vi "JESD Sync TX.vi"(0 "fpga ref in":T7, 2 "txjesd.LmfcDly":fxp<+,5,5>=2.0, 5 "Board Settings in":T1={"VISA resource name"="", "Address Space"=1, "window_offset"=0, "register_addresses"={"MM based Registers"={"Revision"=0, "OldestCompatRev"=0, "signature"=0, "scratch"=0, "LedControl"=0, "BoardHwRev"=0, "BoardControl"=0, "ThermalStatus"=0, "BasebandStatus"=0, "BasebandControl"=0, "BasebandAuxSetup"=0, "BasebandAuxStatus"=0, "LmkSyncOutSetup"=0, " AdcSyncOutSetup"=0, " InjSyncOutSetup"=0, " PxiTrig0OutSetup"=0, " PxiTrig1OutSetup"=0, " PxiTrig2OutSetup"=0, " PxiTrig3OutSetup"=0, " PxiTrig4OutSetup"=0, " PxiTrig5OutSetup"=0, " PxiTrig6OutSetup"=0, " PxiTrig7OutSetup"=0}, "CPLD based Registers"={"SlaveSignature"=0, "SlaveRevision"=0, "SlaveOldestCompatRev"=0, "SlaveScratch"=0, "SlaveSetup"=0, "SlaveStatus"=0, "IDacReg_offset"=0, "LMKRegGrp0_offset"=0, "QDacReg_offset"=0, "BrdTempSensorVal"=0, "TempSensorPowerDown"=0, "GPIOReg_offset"=0, "IAdcReg_offset"=0, "QAdcReg_offset"=0, "LMKRegGrp1_offset"=0, "QadcTempSensorVal"=0, "IadcTempSensorVal"=0, "RevisionReg"=0, "VcxoReg"=0, "CpldStatusReg"=0, "PowerReg"=0, "VBiasEnReg"=0, "ExtRefOeReg"=0, "QdacCtrlReg"=0, "QdacStatusReg"=0, "IdacCtrlReg"=0, "IdacStatusReg"=0, "QdacJtagIn"=0, "QdacJtagOut"=0, "IdacJtagIn"=0, "IdacJtagOut"=0, "IqDcSetupReg"=0, "QadcStatusReg"=0, "IadcStatusReg"=0, "BrdSetupReg"=0, "IqDcRevisionReg"=0, "PllStatusReg"=0, "EndpointScratchReg"=0, "AdcSyncCfgReg"=0, "IqCardOpampReg"=0}, "CPLD Register Offset"=0, "MM  Register Offset"=0, " PxiTrig0OutSetup"=0}, "required_MM_fpga_version"={"signature"=0, "hardware"=0, "current revision"=0, "oldest revision"=0}, "CPLD Oldest Compat Version "={"hardware"=0, "CPLD firmware"=0}, "MM_FPGA_image_location"="", "is_init"=FALSE, "card_type"=enum."ADC", "DacLmkConfigFileName"="", "AdcLmkConfigFileName"="", "AdcConfigFileName"="", "DacConfigFileName_RevA"="", "DacConfigFileName_RevB"="", "Mulde hardware revision"=0, "bypass DAC PLL\n"=FALSE, "IQ Card Revision"=enum."RevA", "board capability"={"baseband sync"=enum."no baseband sync"}} {"Address Space" items=["VXI/VME A16"=1, "VXI/VME A24"=2, "VXI/VME A32"=3, "VXI/VME A64"=4, "PXI Memory Allocations"=9, "PXI Configuration"=10, "PXI BAR0"=11, "PXI BAR1"=12, "PXI BAR2"=13, "PXI BAR3"=14, "PXI BAR4"=15, "PXI BAR5"=16]}, 11 "error in (no error)":errorcluster) -> (4 "fpga ref out":T7, 6 "Board Settings out":T1={"VISA resource name"="", "Address Space"=0, "window_offset"=0, "register_addresses"={"MM based Registers"={"Revision"=0, "OldestCompatRev"=0, "signature"=0, "scratch"=0, "LedControl"=0, "BoardHwRev"=0, "BoardControl"=0, "ThermalStatus"=0, "BasebandStatus"=0, "BasebandControl"=0, "BasebandAuxSetup"=0, "BasebandAuxStatus"=0, "LmkSyncOutSetup"=0, " AdcSyncOutSetup"=0, " InjSyncOutSetup"=0, " PxiTrig0OutSetup"=0, " PxiTrig1OutSetup"=0, " PxiTrig2OutSetup"=0, " PxiTrig3OutSetup"=0, " PxiTrig4OutSetup"=0, " PxiTrig5OutSetup"=0, " PxiTrig6OutSetup"=0, " PxiTrig7OutSetup"=0}, "CPLD based Registers"={"SlaveSignature"=0, "SlaveRevision"=0, "SlaveOldestCompatRev"=0, "SlaveScratch"=0, "SlaveSetup"=0, "SlaveStatus"=0, "IDacReg_offset"=0, "LMKRegGrp0_offset"=0, "QDacReg_offset"=0, "BrdTempSensorVal"=0, "TempSensorPowerDown"=0, "GPIOReg_offset"=0, "IAdcReg_offset"=0, "QAdcReg_offset"=0, "LMKRegGrp1_offset"=0, "QadcTempSensorVal"=0, "IadcTempSensorVal"=0, "RevisionReg"=0, "VcxoReg"=0, "CpldStatusReg"=0, "PowerReg"=0, "VBiasEnReg"=0, "ExtRefOeReg"=0, "QdacCtrlReg"=0, "QdacStatusReg"=0, "IdacCtrlReg"=0, "IdacStatusReg"=0, "QdacJtagIn"=0, "QdacJtagOut"=0, "IdacJtagIn"=0, "IdacJtagOut"=0, "IqDcSetupReg"=0, "QadcStatusReg"=0, "IadcStatusReg"=0, "BrdSetupReg"=0, "IqDcRevisionReg"=0, "PllStatusReg"=0, "EndpointScratchReg"=0, "AdcSyncCfgReg"=0, "IqCardOpampReg"=0}, "CPLD Register Offset"=0, "MM  Register Offset"=0, " PxiTrig0OutSetup"=0}, "required_MM_fpga_version"={"signature"=0, "hardware"=0, "current revision"=0, "oldest revision"=0}, "CPLD Oldest Compat Version "={"hardware"=0, "CPLD firmware"=0}, "MM_FPGA_image_location"="", "is_init"=FALSE, "card_type"=enum."ADC", "DacLmkConfigFileName"="", "AdcLmkConfigFileName"="", "AdcConfigFileName"="", "DacConfigFileName_RevA"="", "DacConfigFileName_RevB"="", "Mulde hardware revision"=0, "bypass DAC PLL\n"=FALSE, "IQ Card Revision"=enum."RevA", "board capability"={"baseband sync"=enum."no baseband sync"}} {"Address Space" items=["VXI/VME A16"=1, "VXI/VME A24"=2, "VXI/VME A32"=3, "VXI/VME A64"=4, "PXI Memory Allocations"=9, "PXI Configuration"=10, "PXI BAR0"=11, "PXI BAR1"=12, "PXI BAR2"=13, "PXI BAR3"=14, "PXI BAR4"=15, "PXI BAR5"=16]}, 15 "error out":errorcluster)   [LabVIEW 2019]
uses:
  TypeDefs/Blank FPGA Reference.ctl
  <instrlib>/niMmWave/ni3610 and ni3630/controls/public/Main Settings.ctl
  <vilib>/Instr/_visa.llb/VISA Register Access Address Space.ctl
  <instrlib>/niMmWave/ni3610 and ni3630/controls/public/Register Adresses.ctl
  <instrlib>/niMmWave/ni3610 and ni3630/controls/public/Base Card Type.ctl
  <instrlib>/niMmWave/ni3610 and ni3630/controls/private/IQ Card Revision.ctl
  <instrlib>/niMmWave/ni3610 and ni3630/controls/public/Board Capability.ctl
  TypeDefs/TX FPGA Reference.ctl
  <instrlib>/niMmWave/ni3610 and ni3630/controls/public/Trigger Source.ctl
  <vilib>/Utility/error.llb/Error Cluster From Error Code.vi
  <vilib>/rvi/errors/niLvFpgaAdjustHostInterfaceError.vi
  <vilib>/rvi/interface/nirviReadWriteControl/nirviReadWriteControl.xnode
  <vilib>/rvi/interface/Simulation/niFpgaSimulationCallBeginRW.vi
  <instrlib>/niMmWave/ni3610 and ni3630/ni3610_and_ni3630_Driver_Lib.lvlib
  NiFpgaLv.dll
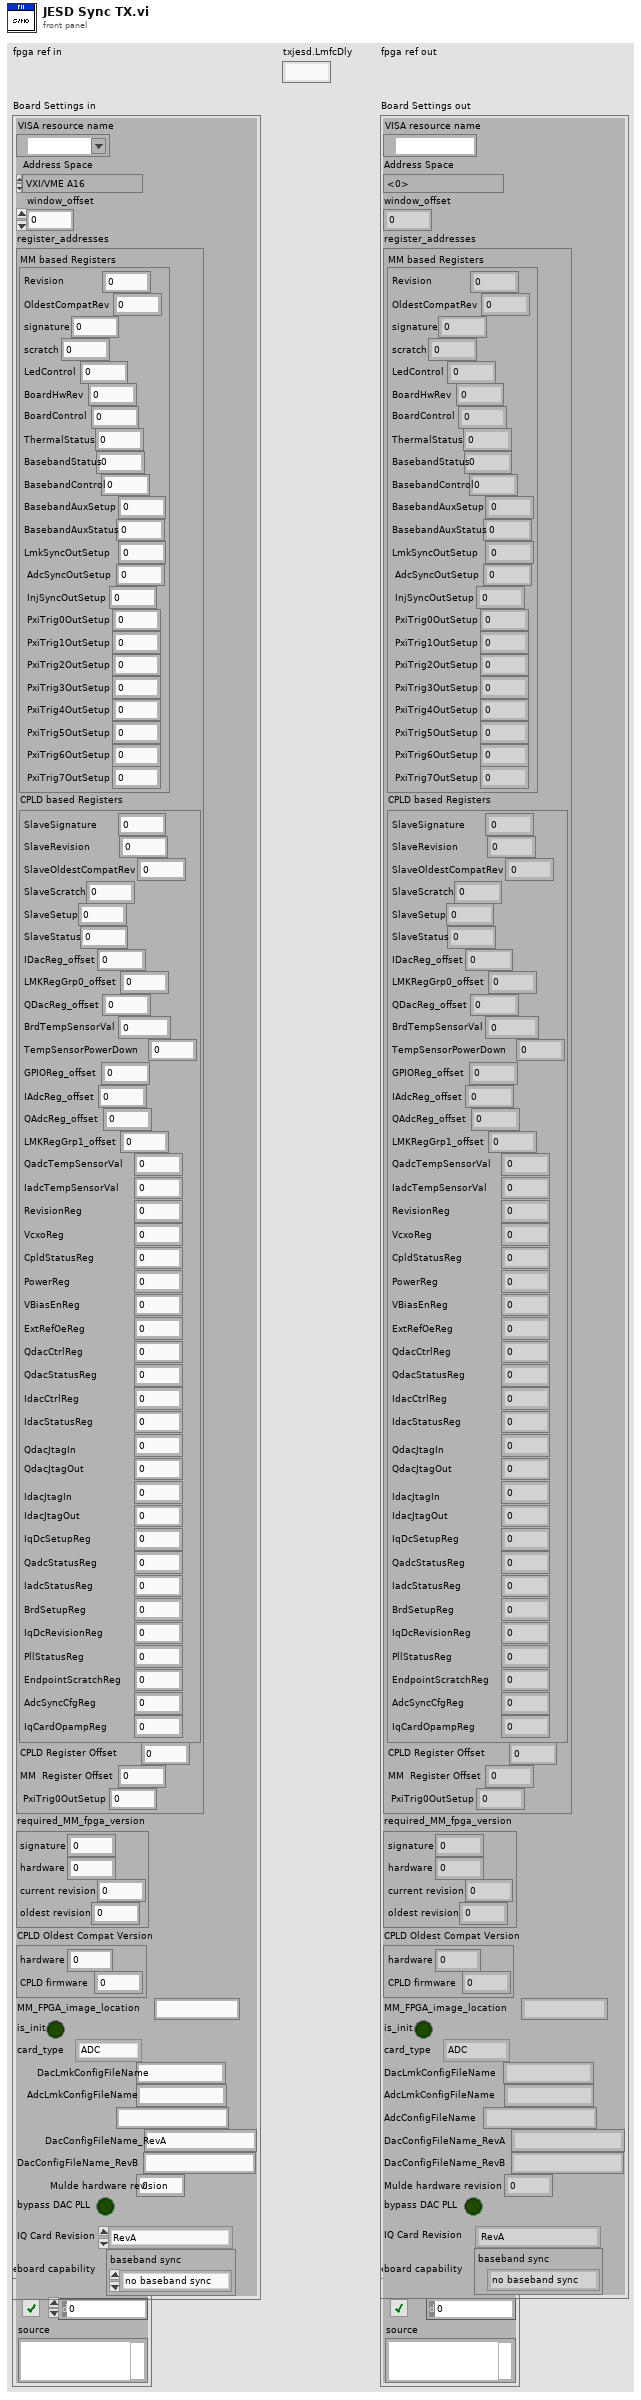
[diagram p1: front panel]
types:
  T1 = typedef "ni3610_and_ni3630_Driver_Lib.lvlib/Main Settings.ctl" = cluster{"VISA resource name":refnum<visa-resource-name>, "Address Space":T2, "window_offset":u32, "register_addresses":T3, "required_MM_fpga_version":cluster{"signature":u32, "hardware":u32, "current revision":u32, "oldest revision":u32}, "CPLD Oldest Compat Version ":cluster{"hardware":u32, "CPLD firmware":u32}, "MM_FPGA_image_location":string, "is_init":bool, "card_type":T4, "DacLmkConfigFileName":string, "AdcLmkConfigFileName":string, "AdcConfigFileName":string, "DacConfigFileName_RevA":string, "DacConfigFileName_RevB":string, "Mulde hardware revision":u8, "bypass DAC PLL\n":bool, "IQ Card Revision":T5, "board capability":T6}
  T2 = typedef "VISA Register Access Address Space.ctl" = u16
  T3 = typedef "ni3610_and_ni3630_Driver_Lib.lvlib/Register Adresses.ctl" = cluster{"MM based Registers":cluster{"Revision":u32, "OldestCompatRev":u32, "signature":u32, "scratch":u32, "LedControl":u32, "BoardHwRev":u32, "BoardControl":u32, "ThermalStatus":u32, "BasebandStatus":u32, "BasebandControl":u32, "BasebandAuxSetup":u32, "BasebandAuxStatus":u32, "LmkSyncOutSetup":u32, " AdcSyncOutSetup":u32, " InjSyncOutSetup":u32, " PxiTrig0OutSetup":u32, " PxiTrig1OutSetup":u32, " PxiTrig2OutSetup":u32, " PxiTrig3OutSetup":u32, " PxiTrig4OutSetup":u32, " PxiTrig5OutSetup":u32, " PxiTrig6OutSetup":u32, " PxiTrig7OutSetup":u32}, "CPLD based Registers":cluster{"SlaveSignature":u32, "SlaveRevision":u32, "SlaveOldestCompatRev":u32, "SlaveScratch":u32, "SlaveSetup":u32, "SlaveStatus":u32, "IDacReg_offset":u32, "LMKRegGrp0_offset":u32, "QDacReg_offset":u32, "BrdTempSensorVal":u32, "TempSensorPowerDown":u32, "GPIOReg_offset":u32, "IAdcReg_offset":u32, "QAdcReg_offset":u32, "LMKRegGrp1_offset":u32, "QadcTempSensorVal":u32, "IadcTempSensorVal":u32, "RevisionReg":u32, "VcxoReg":u32, "CpldStatusReg":u32, "PowerReg":u32, "VBiasEnReg":u32, "ExtRefOeReg":u32, "QdacCtrlReg":u32, "QdacStatusReg":u32, "IdacCtrlReg":u32, "IdacStatusReg":u32, "QdacJtagIn":u32, "QdacJtagOut":u32, "IdacJtagIn":u32, "IdacJtagOut":u32, "IqDcSetupReg":u32, "QadcStatusReg":u32, "IadcStatusReg":u32, "BrdSetupReg":u32, "IqDcRevisionReg":u32, "PllStatusReg":u32, "EndpointScratchReg":u32, "AdcSyncCfgReg":u32, "IqCardOpampReg":u32}, "CPLD Register Offset":u32, "MM  Register Offset":u32, " PxiTrig0OutSetup":u32}
  T4 = typedef "ni3610_and_ni3630_Driver_Lib.lvlib/Base Card Type.ctl" = enum16{"unspecified", "ADC", "DAC"}
  T5 = typedef "ni3610_and_ni3630_Driver_Lib.lvlib/IQ Card Revision.ctl" = enum16{"RevA", "RevB", "RevC", "RevD"}
  T6 = typedef "ni3610_and_ni3630_Driver_Lib.lvlib/Board Capability.ctl" = cluster{"baseband sync":enum16{"no baseband sync", "baseband sync"}}
  T7 = typedef "Blank FPGA Reference.ctl" = refnum<k20>
  T8 = typedef "ni3610_and_ni3630_Driver_Lib.lvlib/Trigger Source.ctl" = enum16{"CntrlDisabled", "LmkSysRef ", "LmkDevClk", "OrDacSync ", "AndDacSync ", "IDacSync", "QDacSync "}
  T9 = typedef "TX FPGA Reference.ctl" = refnum<k20>
  T10 = cluster{"reset":bool, "gtx enable":bool, "jesd enable":bool, "sw sync":bool, "gtx post cursor":fxp<+,5,5>, "gtx pre cursor":fxp<+,5,5>, "gtx diff control":fxp<+,4,4>, "clock enable":bool, "lmfc delay":fxp<+,5,5>, "sysref enable":bool, "sync enable":bool, "trig7 listen":bool, "trig7 invert":bool, "clear data in error":bool}
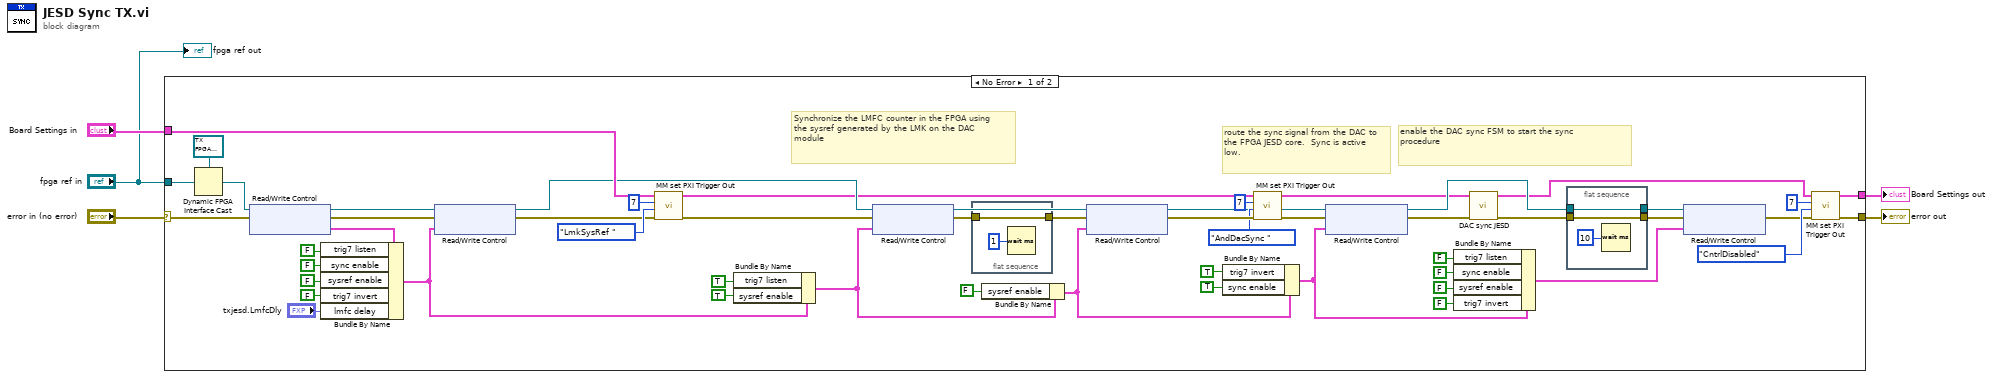
[diagram p0: block diagram]
diagram:
  n1 = case shown="No Error" "error in (no error)" {
    selector: "error in (no error)" -> [w27 w65]
    tunnel: "fpga ref in" -> [w57 _]
    tunnel: [w56 w65] -> w5
    tunnel: "Board Settings in" -> [w55 w64]
    tunnel: [w54 w64] -> w2
    frame No Error {
      # "enable the DAC sync FSM to start the sync procedure"
      # "route the sync signal from the DAC to the FPGA JESD core.  Sync is active low."
      # "Synchronize the LMFC counter in the FPGA using the sysref generated by the LMK on the DAC module"
      n2 = Dynamic FPGA Interface Cast(Session In=T9 refnum ("Refnum in"), Type=w57) -> (Session Out=w29:T9)
      n3 = xnode "Read/Write Control"("FPGA VI Reference In"=w29, "error in"=w27) -> ("FPGA VI Reference Out"=w28:T9, "error out"=w26:errorcluster, "txjesd.control"=w25:T10)
      n4 = Bundle By Name(cluster=w25, "trig7 listen"=FALSE ("trig7.invert"), "sync enable"=FALSE ("txjesd.sync enable"), "sysref enable"=FALSE ("txjesd.sysref enable"), "trig7 invert"=FALSE ("trig7.invert"), "lmfc delay"="txjesd.LmfcDly") -> (w19:T10)
      n5 = xnode "Read/Write Control"("FPGA VI Reference In"=w28, "error in"=w26, "txjesd.control"=w19) -> ("FPGA VI Reference Out"=w42:T9, "error out"=w51:errorcluster)
      n6 = call <instrlib>:"MM set PXI Trigger Out.vi"("error in"=w51, "Trigger Source"=Trigger_Source."LmkSysRef ", "PXI Trigger Select (0..7)"=u8 7, "Board Settings in"=w55) -> ("error out"=w30:errorcluster, "Board Settings out"=w31:T1)  [unwired: 6 in]
      n7 = Bundle By Name(cluster=w19, "trig7 listen"=TRUE ("trig7.listen"), "sysref enable"=TRUE ("txjesd.sysref enable")) -> (w15:T10)
      n8 = xnode "Read/Write Control"("FPGA VI Reference In"=w42, "error in"=w30, "txjesd.control"=w15) -> ("FPGA VI Reference Out"=w36:T9, "error out"=w38:errorcluster)
      n9 = flat-sequence {
        tunnel: w38 -> [w59]
        tunnel: [w59] -> w37
        frame #0 {
          n10 = Wait (ms)(milliseconds to wait=u32 1) -> ()  [unwired: 1 out]
        }
      }
      n11 = Bundle By Name(cluster=w15, "sysref enable"=FALSE ("txjesd.sysref enable")) -> (w14:T10)
      n12 = xnode "Read/Write Control"("FPGA VI Reference In"=w36, "error in"=w37, "txjesd.control"=w14) -> ("FPGA VI Reference Out"=w40:T9, "error out"=w50:errorcluster)
      n13 = Bundle By Name(cluster=w14, "trig7 invert"=TRUE, "sync enable"=TRUE) -> (w7:T10)
      n14 = call <instrlib>:"MM set PXI Trigger Out.vi"("error in"=w50, "Trigger Source"=Trigger_Source."AndDacSync ", "PXI Trigger Select (0..7)"=u8 7, "Board Settings in"=w31) -> ("error out"=w41:errorcluster, "Board Settings out"=w33:T1)  [unwired: 6 in]
      n15 = xnode "Read/Write Control"("FPGA VI Reference In"=w40, "error in"=w41, "txjesd.control"=w7) -> ("FPGA VI Reference Out"=w39:T9, "error out"=w35:errorcluster)
      n16 = Bundle By Name(cluster=w7, "trig7 listen"=FALSE ("trig7.invert"), "sync enable"=FALSE ("txjesd.sync enable"), "sysref enable"=FALSE ("txjesd.sysref enable"), "trig7 invert"=FALSE ("trig7.invert")) -> (w6:T10)
      n17 = call <instrlib>:"DAC sync JESD.vi"("error in"=w35, "Board Settings in"=w33) -> ("error out"=w34:errorcluster, "Board Settings out"=w32:T1)  [unwired: 8 in]
      n18 = flat-sequence {
        tunnel: w39 -> [w62]
        tunnel: w34 -> [w61]
        tunnel: [w62] -> w43
        tunnel: [w61] -> w44
        frame #0 {
          n19 = Wait (ms)(milliseconds to wait=u32 10) -> ()  [unwired: 1 out]
        }
      }
      n20 = xnode "Read/Write Control"("FPGA VI Reference In"=w43, "error in"=w44, "txjesd.control"=w6) -> ("error out"=w45:errorcluster)  [unwired: 1 out]
      n21 = call <instrlib>:"MM set PXI Trigger Out.vi"("error in"=w45, "Trigger Source"=Trigger_Source."CntrlDisabled", "PXI Trigger Select (0..7)"=u8 7, "Board Settings in"=w32) -> ("error out"=w56:errorcluster, "Board Settings out"=w54:T1)  [unwired: 6 in]
    }
    frame Error {
    }
  }
  "error out" <- w5
  "Board Settings out" <- w2
  "fpga ref out" <- "fpga ref in"
